vi "HapticSTM_rawspeed.vi"() -> ()   [LabVIEW 2017]
uses:
  Program Files/National Instruments/LabVIEW 2019/user.lib/HapticSTM/HapticSTM.lvlib
  SubVIs/GlobalClicksHeight_raw.vi
  Program Files/National Instruments/LabVIEW 2019/user.lib/Nanonis Prog Interface V5/Nanonis Prog Interface.lvlib
panel:
  in  "Z Write?":bool
  in  "Save":bool
  in  "# Sample Points":i32=4096
  in  "Version?":bool=TRUE
  in  "Setpoint (pA)":dbl=100.0
  in  "Depth (pA)":dbl=280.0
  in  "Shift (in)":dbl format="%.1f"
  in  "Hardness":dbl=0.7 format="%.1f"
  out "function return":i32
  in  "Scaling?":u16(ring) items=["Medium", "Large", "Small"]
  out "Setpoint (pA)":dbl
  in  "Maximum (pA)":dbl=7000.0
  out "Filtered Current (pA)":dbl format="%.1f"
  out "Current (pA)":dbl format="%.1f"
  out "Oy":dbl
  out "Ox":dbl
  out "W":dbl
  out "H":dbl
  out "Z Write":dbl format="%^.1e"
  in  "Planing?":bool
  out "Button":bool
  out "Fy":dbl format="%.1f"
  out "Fz":dbl format="%.1f"
  out "Fx":dbl format="%.1f"
  out "x":dbl format="%.1f"
  out "y":dbl format="%.1f"
  out "z":dbl format="%0.1f"
  in  "Mode":u16(ring) items=["Log w/ Exp Z", "Log w/ Lin Z", "Coulomb Force", "Lennard Jones", "r^6"]
  in  "Reset Clicks":bool
  out "Clicks":i32
  in  "STOP":bool
  in  "START":bool
  out "Seq":i32
  out "SeqString":string
  out "Raw and Scaled Z Positions":T1(graph)
  out "Scaled Force and Current":T2(graph)
  # "Super Ultra Mega Haptic STM Controller 3000"
  # "Haptic Pen"
  # "Nanonis"
  # "Position"
  # "Z Controller"
  # "Force"
  # "Frame"
  # "Surface"
  # "Options"
  # "Addons"
  # "Test Data"
  # "Live"
  # "Current"
  # "No"
  # "Yes"
  # "Planing"
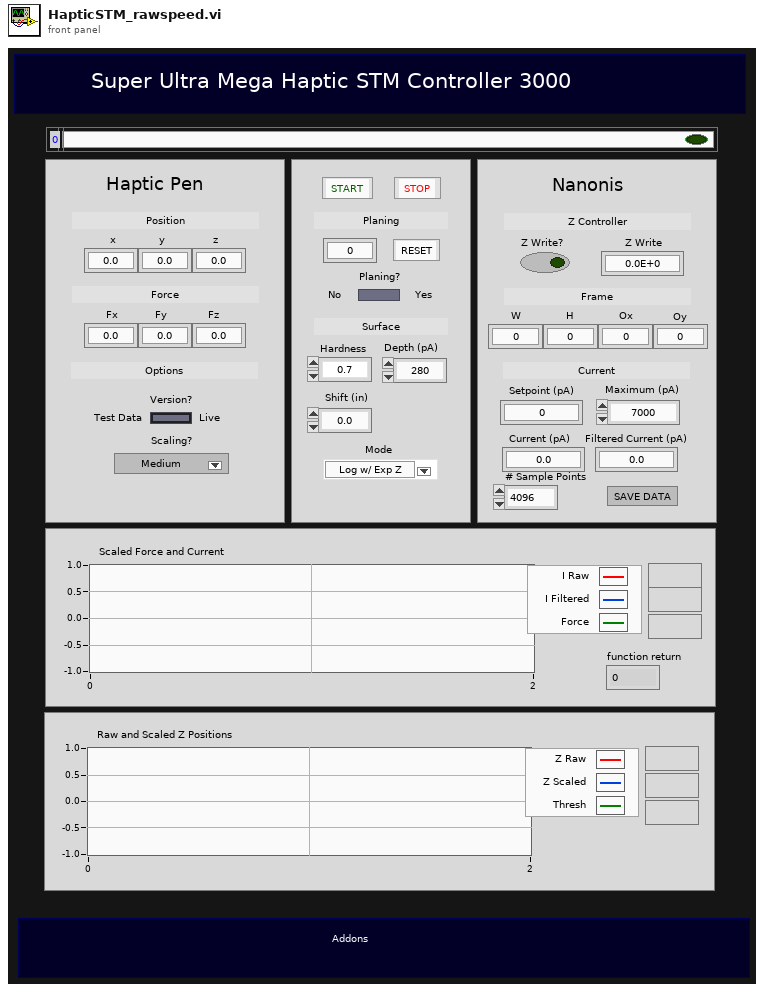
[diagram p1: front panel]
types:
  T1 = cluster{dbl, "function return":dbl, "function return":dbl}
  T2 = cluster{"Current (pA)":dbl, "Filtered Current (pA)":dbl, dbl}
  T3 = cluster{"Size (m)":cluster{"Width":sgl, "Height":sgl}, "Center coordinates (m)":cluster{"Xc":sgl, "Yc":sgl}}
  T4 = cluster{"Z Raw":dbl, "Z scaled":dbl, "threshhold":dbl}
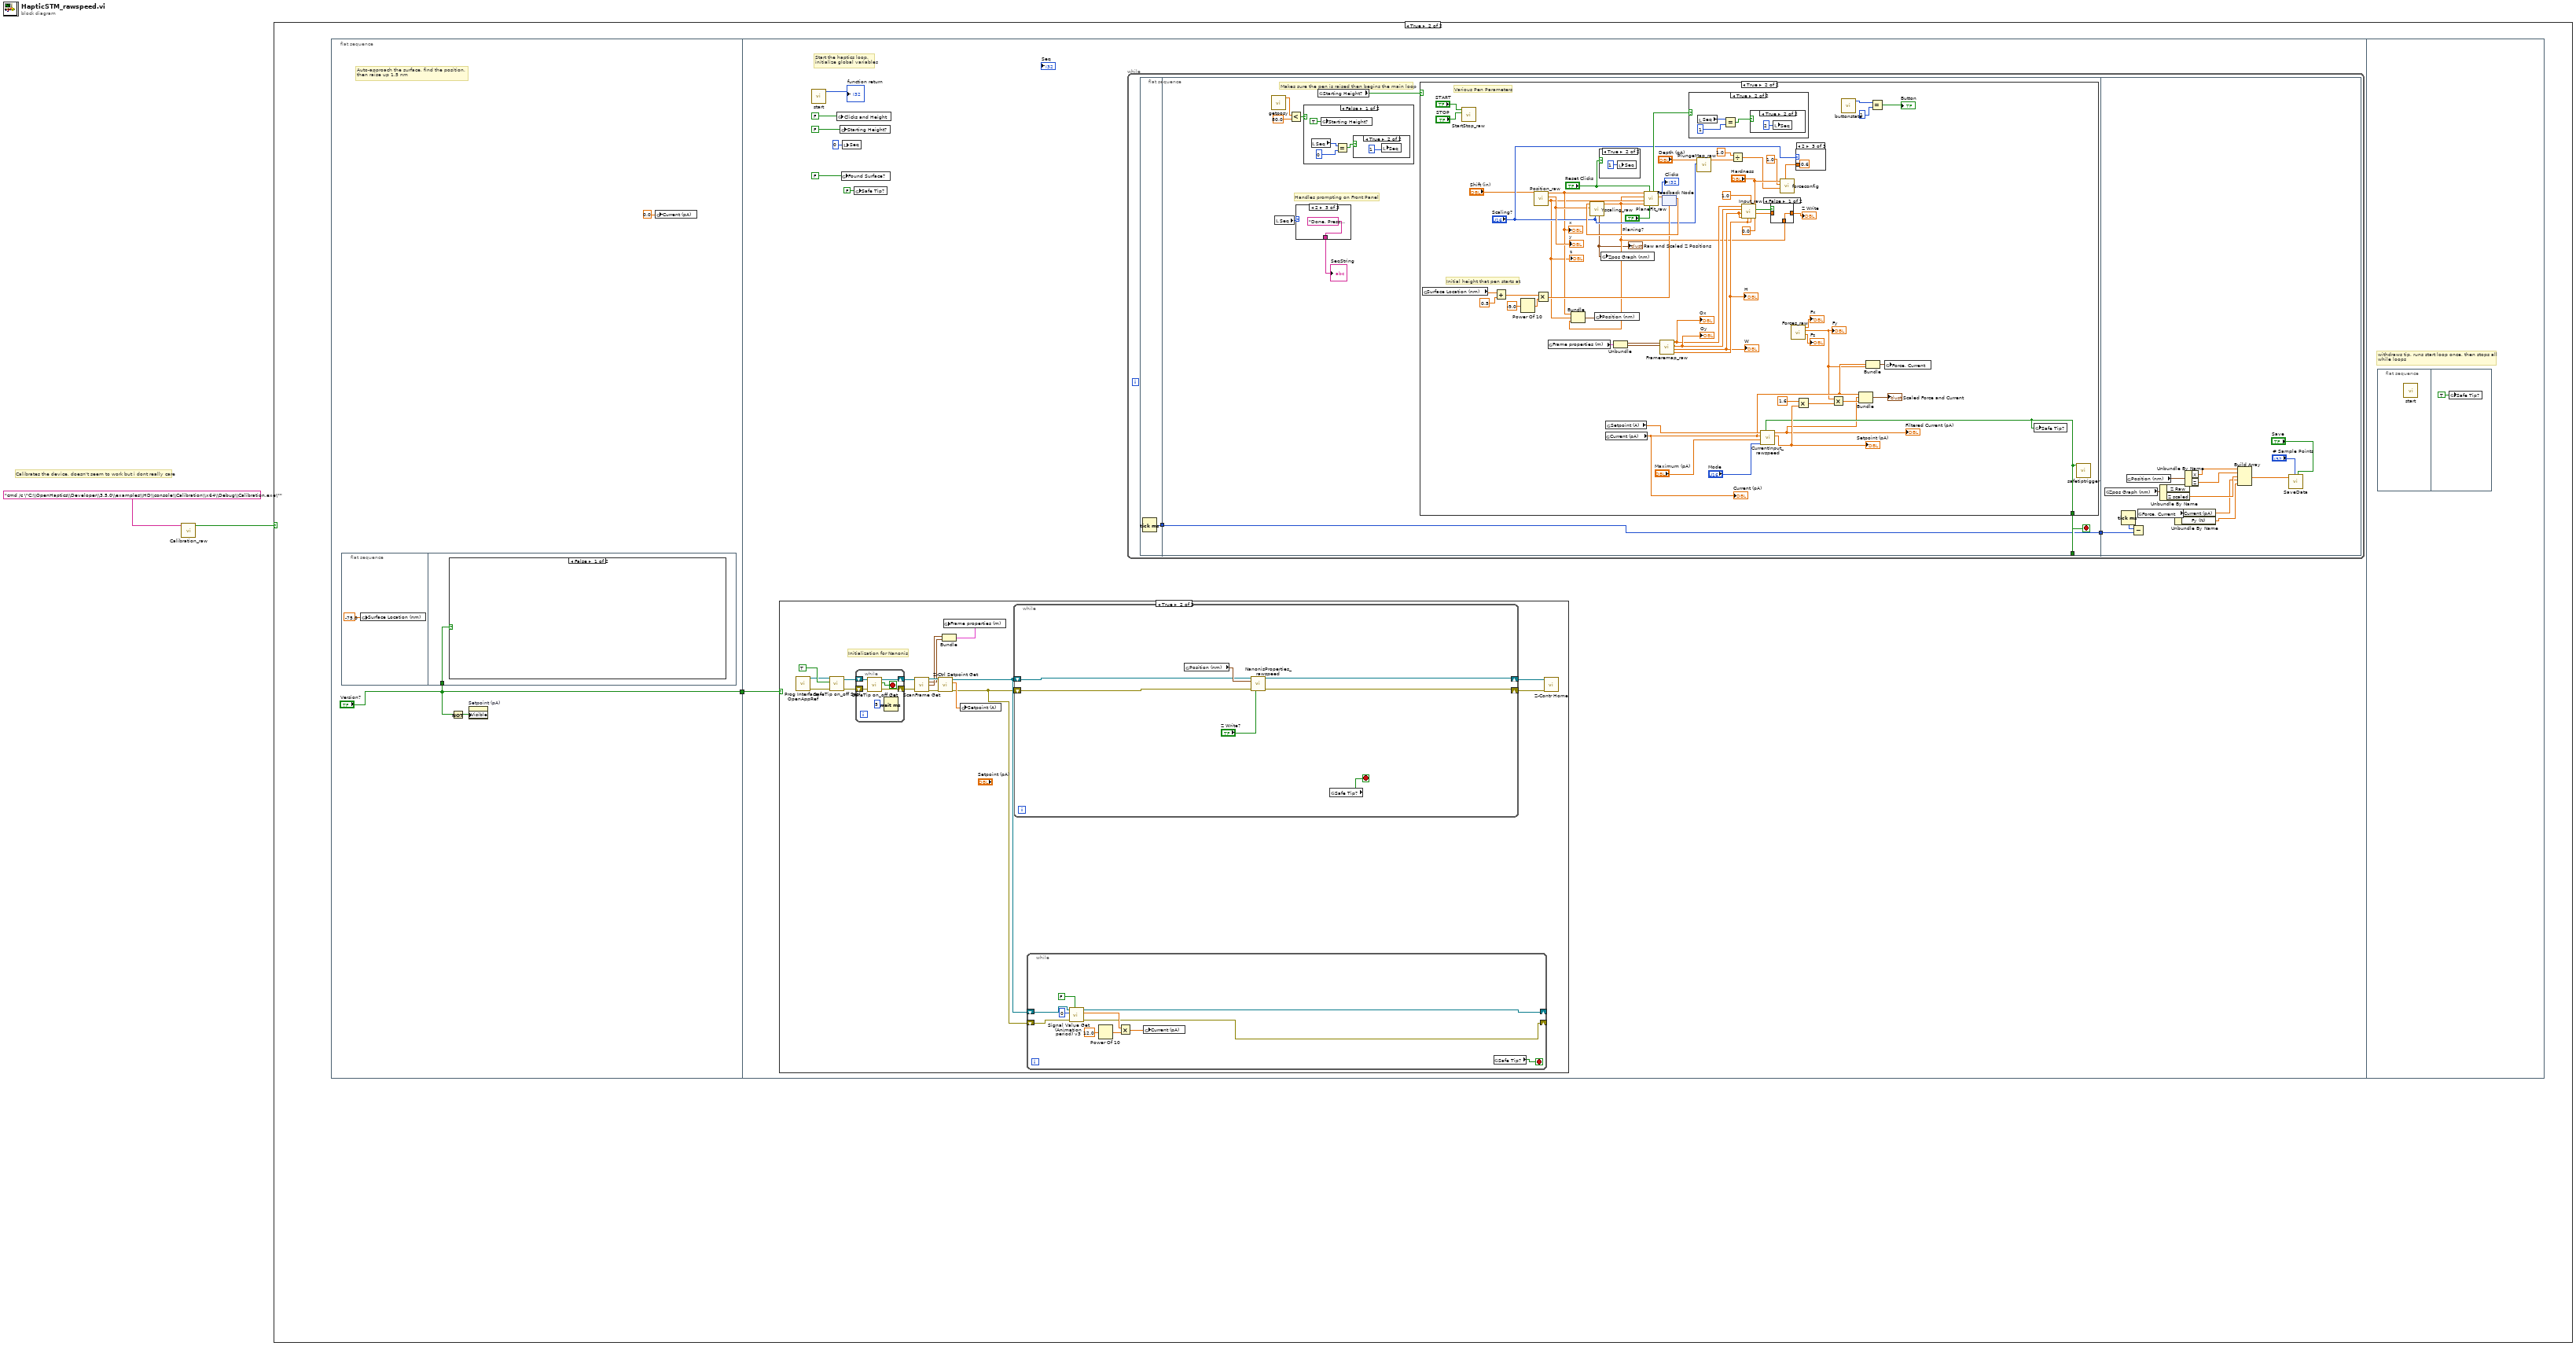
[diagram p0: block diagram]
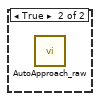
[diagram p3: hidden frame]
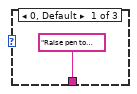
[diagram p5: hidden frame]
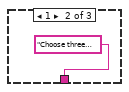
[diagram p6: hidden frame]
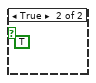
[diagram p8: hidden frame]
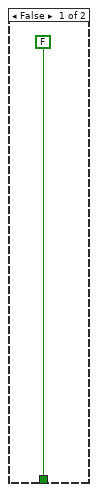
[diagram p9: hidden frame]
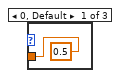
[diagram p10: hidden frame]
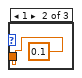
[diagram p11: hidden frame]
diagram:
  # "Calibrates the device, doesn't seem to work but i dont really care"
  n1 = call "Calibration_raw.vi"("command line"="cmd /c \"C:\\OpenHaptics\\Developer\\3.5.0\\examples\\HD\\console\\Calibration\\x64\\Debug\\Calibration.exe\"") -> ("Calibration Complete?"=w2:bool)  [unwired: 10 in]
  n2 = case shown="True" w2 {
    frame False {
    }
    frame True {
      n3 = flat-sequence {
        tunnel: ["Version?"] -> w3
        tunnel: w3 -> [w9]
        frame #0 {
          # "Auto-approach the surface, find the position, \nthen raise up 1.5 nm"
          n4 = flat-sequence {
            tunnel: "Version?" -> [w8]
            frame #0 {
              n5 = global write "GlobalClicksHeight_raw.vi" "Surface Location (nm)"(-75.0 ("Surface Location")) -> ()
            }
            frame #1 {
              n6 = case shown="False" w8 {
                frame False {
                }
                frame True {
                  n7 = call "AutoApproach_raw.vi"() -> ()  [unwired: 12 in]
                }
              }
            }
          }
          n8 = Not(x="Version?") -> (.not. x?=w5:bool)
          n9 = property on="Setpoint (pA)" class="DigNum (strict)"("Visible"=w5) -> ()  [unwired: 2 in, 2 out]
          n10 = global write "GlobalClicksHeight_raw.vi" "Current (pA)"(0.0 ("Current (pA)")) -> ()
        }
        frame #1 {
          # "Start the haptics loop,\ninitialize global variables"
          n11 = case shown="True" w9 {
            frame False {
            }
            frame True {
              # "Initialization for Nanonis"
              n12 = call <userlib>:"Prog Interface - OpenAppRef.vi"() -> ("Error out"=w30:errorcluster, "Application reference"=w31:refnum<vi>)  [unwired: 6 in]
              n13 = call <userlib>:"SafeTip on_off Set.vi"("error in (no error)"=w30, "SafeTip ON/OFF"=TRUE, "Application ref in"=w31) -> ("error out"=w28:errorcluster, "Application ref out"=w29:refnum<vi>)  [unwired: 7 in]
              n14 = while {
                shift-right: [w46] -> w27
                shift-left: w29 -> [w48]
                shift-right: [w45] -> w26
                shift-left: w28 -> [w47]
                stop <- w49 stop-if-true
                n15 = call <userlib>:"SafeTip on_off Get.vi"("error in (no error)"=w47, "Application ref in"=w48) -> ("error out"=w45:errorcluster, "SafeTip on/off status"=w49:bool, "Application ref out"=w46:refnum<vi>)  [unwired: 7 in]
                n16 = Wait (ms)(milliseconds to wait=u32 5) -> ()  [unwired: 1 out]
              }
              n17 = call <userlib>:"ScanFrame Get.vi"("Application ref in"=w27, "error in (no error)"=w26) -> ("Application ref out"=w25:refnum<vi>, "Center coordinates (m)"=w18:cluster{"Xc":sgl, "Yc":sgl}, "Size (m)"=w19:cluster{"Width":sgl, "Height":sgl}, "error out"=w24:errorcluster)  [unwired: 9 in, 1 out]
              n18 = call <userlib>:"Z-Ctrl Setpoint Get.vi"("error in (no error)"=w24, "Application ref in"=w25) -> ("error out"=w16:errorcluster, "Z Controller setpoint"=w23:sgl, "Application ref out"=w17:refnum<vi>)  [unwired: 6 in]
              n19 = Bundle("Size (m)"=w19, "Center coordinates (m)"=w18) -> (w20:T3)  [unwired: 1 in]
              n20 = global write "GlobalClicksHeight_raw.vi" "Frame properties (m)"(w20) -> ()
              n21 = global write "GlobalClicksHeight_raw.vi" "Setpoint (A)"(w23) -> ()
              n22 = while {
                shift-right: [w50] -> w21
                shift-left: w16 -> [w52]
                shift-right: [w51] -> w22
                shift-left: w17 -> [w53]
                stop <- w56 stop-if-true
                n23 = global read "GlobalClicksHeight_raw.vi" "Position (nm)"() -> (w54:cluster{"X":dbl, "Z":dbl, "Y":dbl})
                n24 = call "NanonisProperties_rawspeed.vi"("Application ref in"=w53, "Position (nm)"=w54, "error in (no error)"=w52, "Z Write?"="Z Write?") -> ("Application ref out"=w51:refnum<vi>, "error out"=w50:errorcluster)  [unwired: 10 in]
                n25 = global read "GlobalClicksHeight_raw.vi" "Safe Tip?"() -> (w56:bool)
              }
              n26 = while {
                shift-right: [w34] -> _
                shift-left: w16 -> [w36]
                shift-right: [w35] -> _
                shift-left: w17 -> [w37]
                stop <- w43 stop-if-true
                n27 = call <userlib>:"Signal Value Get (Animation period) v3.vi"("Wait for newest data (F=False)"=FALSE, "error in (no error)"=w36, "Signal index (0-127)"=i8 0, "Application ref in"=w37) -> ("error out"=w34:errorcluster, "Signal value"=w38:sgl, "Application ref out"=w35:refnum<vi>)  [unwired: 4 in]
                n28 = Power Of 10(x=12.0) -> (10^x=w41:dbl)
                n29 = Multiply(x=w38, y=w41) -> (x*y=w40:dbl)
                n30 = global write "GlobalClicksHeight_raw.vi" "Current (pA)"(w40) -> ()
                n31 = global read "GlobalClicksHeight_raw.vi" "Safe Tip?"() -> (w43:bool)
              }
              n32 = call <userlib>:"Z-Contr Home.vi"("Error in (no error)"=w21, "Application ref in"=w22) -> ()  [unwired: 8 in, 2 out]
            }
          }
          n33 = call "start.vi"() -> ("function return"=→"function return":i32)  [unwired: 11 in]
          n34 = global write "GlobalClicksHeight_raw.vi" "Clicks and Height"(FALSE ("Clicks and Height")) -> ()
          n35 = global write "GlobalClicksHeight_raw.vi" "Starting Height?"(FALSE ("Clicks and Height")) -> ()
          n36 = global write "GlobalClicksHeight_raw.vi" "Found Surface?"(FALSE ("Clicks and Height")) -> ()
          n37 = local write "Seq"(0 ("Seq")) -> ()
          n38 = global write "GlobalClicksHeight_raw.vi" "Safe Tip?"(FALSE ("Safe Tip?")) -> ()
          n39 = while {
            stop <- w59 stop-if-true
            n40 = flat-sequence {
              tunnel: [w60] -> w58
              tunnel: [w62] -> w59
              tunnel: w58 -> [w61]
              tunnel: [w61] -> w57
              tunnel: w57 -> [w158]
              frame #0 {
                n41 = Tick Count (ms)() -> (millisecond timer value=w60:u32)
              }
              frame #1 {
                # "Makes sure the pen is raised then begins the main loop"
                # "Handles prompting on Front Panel"
                n42 = call "getposy.vi"() -> ("function return"=w68:dbl)  [unwired: 11 in]
                n43 = local read "Seq"() -> (w64:i32)
                n44 = Less?(x=w68, y=80.0) -> (x < y?=w66:bool)
                n45 = case shown="2" w64 {
                  tunnel: ["Raise pen to begin." "Choose three points, then raise the arm to plane." "Done. Press 'STOP' to stop at anytime."] -> w63
                  frame 0, Default {
                  }
                  frame 1 {
                  }
                  frame 2 {
                  }
                }
                "SeqString" <- w63
                n46 = case shown="False" w66 {
                  frame False {
                    n47 = local read "Seq"() -> (w74:i32)
                    n48 = global write "GlobalClicksHeight_raw.vi" "Starting Height?"(TRUE ("Starting Height?")) -> ()
                    n49 = Equal?(x=w74, y=0) -> (x = y?=w72:bool)
                    n50 = case shown="True" w72 {
                      frame False {
                      }
                      frame True {
                        n51 = local write "Seq"(1 ("Seq")) -> ()
                      }
                    }
                  }
                  frame True {
                    (unwired) TRUE ("Clicks and Height")
                  }
                }
                n52 = global read "GlobalClicksHeight_raw.vi" "Starting Height?"() -> (w65:bool)
                n53 = case shown="True" w65 {
                  tunnel: [FALSE ("Current Maxed?") w87] -> w62
                  frame False {
                  }
                  frame True {
                    # "Initial height that pen starts at"
                    # "Various Pen Parameters"
                    n54 = global read "GlobalClicksHeight_raw.vi" "Surface Location (nm)"() -> (w101:dbl)
                    n55 = call "StartStop_raw.vi"("STOP"="STOP", "START"="START") -> ()  [unwired: 10 in]
                    n56 = Add(x=w101, y=0.5) -> (x+y=w98:dbl)
                    n57 = Power Of 10(x=-9.0) -> (10^x=w97:dbl)
                    n58 = call "Position_raw.vi"("Shift"="Shift (in)") -> ("Z"=w90:dbl, "Y"=w126:dbl, "X"=w91:dbl)  [unwired: 8 in]
                    "x" <- w91
                    "y" <- w126
                    "z" <- w90
                    n59 = Multiply(x=w98, y=w97) -> (x*y=w99:dbl)
                    n60 = global read "GlobalClicksHeight_raw.vi" "Frame properties (m)"() -> (w86:cluster{cluster{dbl, dbl}, cluster{dbl, dbl}})
                    n61 = case shown="True" "Reset Clicks" {
                      frame False {
                      }
                      frame True {
                        n62 = local write "Seq"(1 ("Seq")) -> ()
                      }
                    }
                    n63 = global read "GlobalClicksHeight_raw.vi" "Current (pA)"() -> (w81:dbl)
                    "Current (pA)" <- w81
                    n64 = global read "GlobalClicksHeight_raw.vi" "Setpoint (A)"() -> (w88:dbl)
                    n65 = Unbundle(w86) -> (w85:cluster{dbl, dbl}, w84:cluster{dbl, dbl})
                    n66 = call "Frameremap_raw.vi"("Frame Origin (m)"=w84, "Frame Size (m)"=w85) -> ("FH (nm)"=w111:dbl, "FW (nm)"=w110:dbl, "Z Origin (nm)"=w109:dbl, "X Origin (nm)"=w108:dbl)  [unwired: 6 in]
                    "H" <- w111
                    "W" <- w110
                    "Ox" <- w108
                    "Oy" <- w109
                    n67 = feedback #1(w99) -> (w130:dbl)
                    n68 = call "Yscaling_raw.vi"("Scaling?"="Scaling?", "Y"=w126, "Plane Height (m)"=w130) -> ("y scaled (m)"=w89:dbl, "Zpos Graph (nm)"=w79:T1)  [unwired: 7 in]
                    "Raw and Scaled Z Positions" <- w79
                    n69 = Bundle("X"=w91, "Z"=w90, "y scaled (m)"=w89) -> (w92:cluster{"X":dbl, "Z":dbl, "y scaled (m)":dbl})  [unwired: 1 in]
                    n70 = global write "GlobalClicksHeight_raw.vi" "Position (nm)"(w92) -> ()
                    n71 = global write "GlobalClicksHeight_raw.vi" "Zpos Graph (nm)"(w79) -> ()
                    n72 = call "PlaneFit_raw.vi"("Planing y/n?"="Planing?", "Reset Clicks"="Reset Clicks", "Y PEN"=w89, "Z"=w90, "Nano Z"=w89, "X"=w91) -> ("Plane Height (m)"=w131:dbl, "Clicks"=→"Clicks":i32, "Planing Done?"=w120:bool)  [unwired: 3 in]
                    n73 = feedback-in #1(w131) -> ()
                    n74 = case shown="True" w120 {
                      frame False {
                      }
                      frame True {
                        n75 = local read "Seq"() -> (w145:i32)
                        n76 = Equal?(x=w145, y=1) -> (x = y?=w143:bool)
                        n77 = case shown="True" w143 {
                          frame False {
                          }
                          frame True {
                            n78 = local write "Seq"(2 ("Seq")) -> ()
                          }
                        }
                      }
                    }
                    n79 = call "PlungeMap_raw.vi"("Scaling?"="Scaling?", "Input (pA)"="Depth (pA)") -> ("output"=w102:dbl)  [unwired: 9 in]
                    n80 = Divide(x=1.0, y=w102) -> (x/y=w112:dbl)
                    n81 = call "Input_raw.vi"("Current * 10^input"=0.0, "Sensitivity"="Hardness", "Scopez"=w111, "Drag"=1.0, "FH"=w111, "FW"=w110, "Scopex"=w110, "Z origin"=w109, "X origin"=w108) -> ("Scaled Current"=w114:dbl, "feedback"=w116:bool)  [unwired: 1 in]
                    n82 = call "CurrentInput_rawspeed.vi"("Mode"="Mode", "Maximum (pA)"="Maximum (pA)", "Current (pA)"=w81, "Setpoint (A)"=w88) -> ("Setpoint (pA)"=w104:dbl, "Filtered Current (pA)"=w80:dbl, "Safetip?"=w87:bool)  [unwired: 5 in]
                    "Filtered Current (pA)" <- w80
                    "Setpoint (pA)" <- w104
                    n83 = case shown="False" w116 {
                      tunnel: [w140 w141] -> w115
                      tunnel: w114 -> [_ w141]
                      tunnel: w89 -> [w140 _]
                      frame False {
                      }
                      frame True {
                      }
                    }
                    "Z Write" <- w115
                    n84 = call "Forces_raw.vi"() -> ("Fz"=→"Fz":dbl, "Fy"=w78:dbl, "Fx"=→"Fx":dbl)  [unwired: 9 in]
                    "Fy" <- w78
                    n85 = case shown="2" "Scaling?" {
                      tunnel: [0.5 0.1 0.6] -> w95
                      frame 0, Default {
                      }
                      frame 1 {
                      }
                      frame 2 {
                      }
                    }
                    n86 = call "forceconfig.vi"("spc"=w95, "c"=w112, "b"=1.0, "a"="Hardness") -> ()  [unwired: 8 in]
                    n87 = Multiply(x=1.6 ("y"), y=w104) -> (x*y=w127:dbl)
                    n88 = Multiply(x=w78, y=w127) -> (x*y=w129:dbl)
                    n89 = call "buttonstate.vi"() -> ("function return"=w125:i32)  [unwired: 11 in]
                    n90 = Bundle("Current (pA)"=w81, "Filtered Current (pA)"=w80, w129) -> (→"Scaled Force and Current":T2)  [unwired: 1 in]
                    n91 = Bundle("Current (pA)"=w81, "Fy"=w78) -> (w82:cluster{"Current (pA)":dbl, "Fy":dbl})  [unwired: 1 in]
                    n92 = Equal?(x=w125, y=1) -> (x = y?=→"Button":bool)
                    n93 = global write "GlobalClicksHeight_raw.vi" "Force, Current"(w82) -> ()
                    n94 = global write "GlobalClicksHeight_raw.vi" "Safe Tip?"(w87) -> ()
                    n95 = call "safetiptrigger.vi"("triggered"=w87) -> ()  [unwired: 11 in]
                  }
                }
              }
              frame #2 {
                n96 = global read "GlobalClicksHeight_raw.vi" "Zpos Graph (nm)"() -> (w154:T4)
                n97 = Tick Count (ms)() -> (millisecond timer value=w159:u32)
                n98 = global read "GlobalClicksHeight_raw.vi" "Position (nm)"() -> (w157:cluster{"X":dbl, "Z":dbl, "Y":dbl})
                n99 = Subtract(x=w159, y=w158) -> ()  [unwired: 1 out]
                n100 = global read "GlobalClicksHeight_raw.vi" "Force, Current"() -> (w152:cluster{"Current (pA)":dbl, "Fy (N)":dbl})
                n101 = Unbundle By Name(w154) -> ("Z scaled"=w153:dbl)  [unwired: 1 out]
                n102 = Unbundle By Name(w152) -> ("Current (pA)"=w151:dbl, "Fy (N)"=w150:dbl)
                n103 = Unbundle By Name(w157) -> ("X"=w156:dbl, "Z"=w155:dbl)
                n104 = Build Array(w156, w155, w153, w151, w150) -> (w149:dbl[])
                n105 = call "SaveData.vi"("Save"="Save", "# Sample Points"="# Sample Points", "Data"=w149) -> ()  [unwired: 9 in]
              }
            }
          }
        }
        frame #2 {
          # "withdraws tip, runs start loop once, then stops all\nwhile loops"
          n106 = flat-sequence {
            frame #0 {
              n107 = call "start.vi"() -> ()  [unwired: 11 in, 1 out]
            }
            frame #1 {
              n108 = global write "GlobalClicksHeight_raw.vi" "Safe Tip?"(TRUE ("Safe Tip?")) -> ()
            }
          }
        }
      }
    }
  }
